vi "4_5 Construct a VI Pro2.vi"() -> ()   [LabVIEW 2025]
panel:
  in  "stop":bool
  out "Integer":bool
  in  "Floating Point":dbl
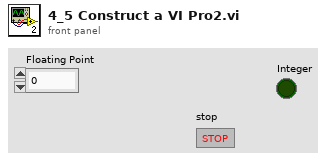
[diagram p1: front panel]
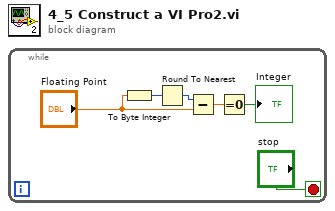
[diagram p0: block diagram]
diagram:
  n1 = while {
    stop <- "stop" stop-if-true
    n2 = To Byte Integer(number="Floating Point") -> (8bit integer=w5:i8)
    n3 = Round To Nearest(number=w5) -> (nearest integer value=w6:i8)
    n4 = Subtract(x=w6, y="Floating Point") -> (x-y=w3:dbl)
    n5 = Equal To 0?(x=w3) -> (x = 0?=→"Integer":bool)
  }
